vi "PQsetErrorVerbosity.vi"(8 "error in (no error)":errorcluster, 10 "verbosity":i32) -> (0 "error out":errorcluster, 2 "PGVerbosity":i32)   [LabVIEW 2019, in "libpqlv64.lvlib"]
uses:
  libpqlv64.lvlib
  libpq.dll
panel:
  in  "conn":u32
  out "conn_out":u32
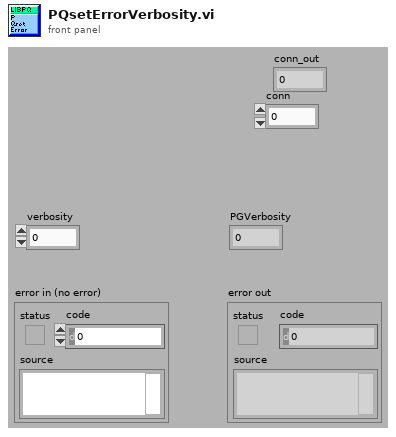
[diagram p1: front panel]
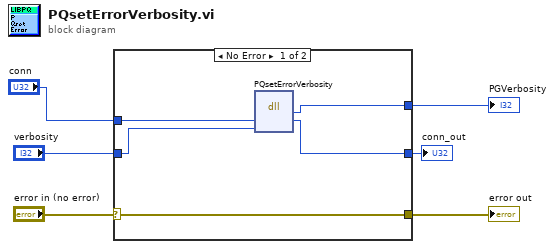
[diagram p0: block diagram]
diagram:
  n1 = case shown="No Error" "error in (no error)" {
    selector: "error in (no error)" -> [w11 w13]
    tunnel: [w11 w13] -> w5
    tunnel: [w10 _] -> w4
    tunnel: [w9 w12] -> w2
    tunnel: "verbosity" -> [w8 _]
    tunnel: "conn" -> [w7 w12]
    frame No Error {
      n2 = dll-call lib="libpq.*" fn="PQsetErrorVerbosity"("conn"=w7, "verbosity"=w8) -> ("PQVerbosity"=w10:i32, "conn"=w9:u32)  [unwired: 4 in, 2 out]
    }
    frame Error {
    }
  }
  "PGVerbosity" <- w4
  "error out" <- w5
  "conn_out" <- w2
